vi "DelayBetweenSquares.vi"() -> (2 "milliseconds to wait":u32)   [LabVIEW 2020]
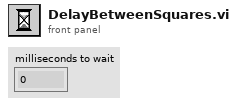
[diagram p1: front panel]
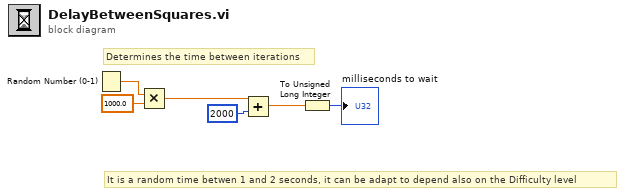
[diagram p0: block diagram]
diagram:
  # "It is a random time betwen 1 and 2 seconds, it can be adapt to depend also on the Difficulty level"
  # "Determines the time between iterations"
  n1 = Random Number (0-1)() -> (number: 0 to 1=w6:dbl)
  n2 = Multiply(x=w6, y=1000.0) -> (x*y=w4:dbl)
  n3 = Add(x=w4, y=u32 2000 ("milliseconds to wait")) -> (x+y=w1:dbl)
  n4 = To Unsigned Long Integer(number=w1) -> (unsigned 32bit integer=→"milliseconds to wait":u32)
